vi "Check if Measurement Ready.vi"(8 "error in (no error)":errorcluster) -> (0 "error out":errorcluster)   [LabVIEW 2019]
uses:
  Global Operations.ctl
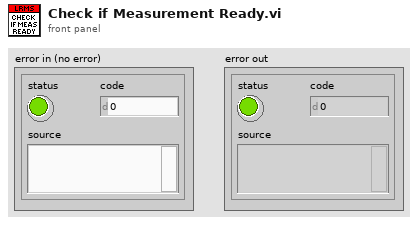
[diagram p1: front panel]
types:
  T1 = typedef "Global Operations.ctl" = enum16{"Get", "Set"}
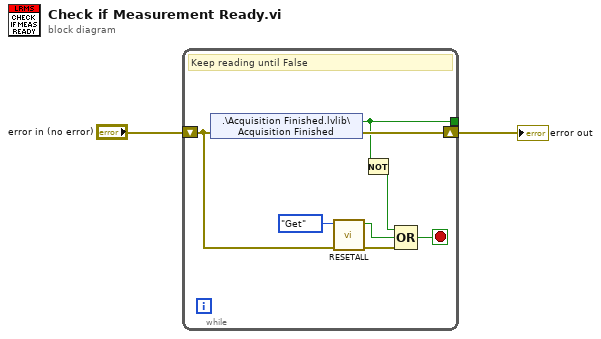
[diagram p0: block diagram]
diagram:
  n1 = while {
    shift-right: [w10] -> w1
    shift-left: "error in (no error)" -> [w5]
    tunnel: [w9] -> _
    stop <- w3 stop-if-true
    # "Keep reading until False"
    n2 = shared-variable ".\\Acquisition Finished.lvlib\\Acquisition Finished"(error in=w5) -> (w9:bool, error out=w10:errorcluster)
    n3 = call "RESETALL.vi"("error in (no error)"=w5, "Operation"=Global_Operations."Get") -> ("error out"=w7:errorcluster, "RESETALL?"=w6:bool)  [unwired: 8 in]
    n4 = Not(x=w9) -> (.not. x?=w4:bool)
    n5 = Compound Arithmetic op=OR(w4, w6, w7) -> (w3:bool)
  }
  "error out" <- w1
